vi "run.vi"(8 "error in (no error)":errorcluster, 11 "GenericExperiment in":refnum<class "ExperimentControllerDL090430DAQmxTriggered.lvclass">) -> (0 "error out":errorcluster, 3 "GenericExperiment out":refnum<class "ExperimentControllerDL090430DAQmxTriggered.lvclass">)   [LabVIEW 2010, in "ExperimentControllerDL090430DAQmxTriggered.lvclass"]
uses:
  ExperimentControllerDL090430DAQmxTriggered.lvclass
  internal_trigger_enum.ctl
  main/labview_source/controls/undock_button.ctl
  common/enumerations/top-level_component_type_enum.ctl
  state_enum.ctl
  ExperimentControllerDL090430DAQmxTriggered.lvclass/ExperimentControllerDL090430DAQmxTriggered.ctl
  main/labview_source/type_definitions/enumerations/main_trigger_enum.ctl
  GenericExperimentController/GenericExperimentController/GenericExperimentController.lvclass
  wait_for_enum.ctl
  common/classes/ErrorController/ErrorController/class_data.vi
  common/classes/ErrorController/ErrorController/ErrorController.lvclass
panel:
  in  "button:undock":T1
  in  "Tab Control":enum32{"User", "Debug", "About"}(tab)
  out "current sweep no.":i32
  out "last trigger":T2
  out "statemachine loop counter":i32
  out "last action":T2
  out "sender":T3=enum."ImagingMode"
  out "event loop error":errorcluster
  out "statemachine loop error":errorcluster
  out "finished?":bool
  out "state":T4
  # "With this experiment controller, each sweep is triggered by a TTL trigger."
  # "DL090430TriggeredExperimentController\n\nImplemented by:\nDominik Langer, University of Zurich, Switzerland\nMarcel van 't Hoff, University of Zurich, Switzerland"
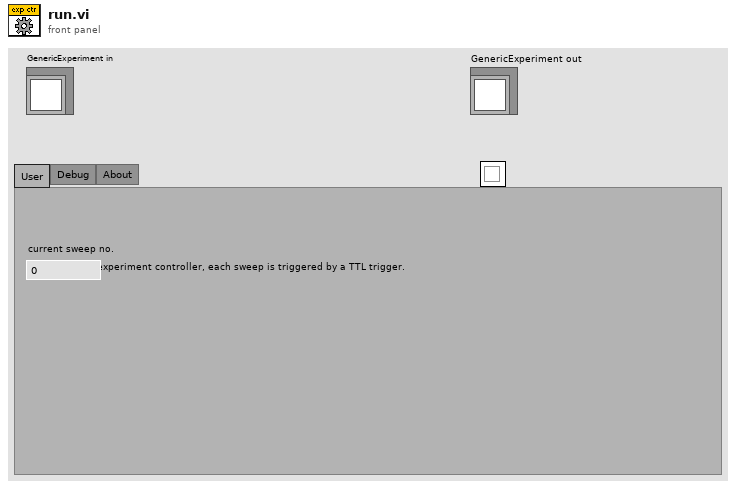
[diagram p1: front panel]
types:
  T1 = typedef "undock_button.ctl" = bool
  T2 = typedef "ExperimentControllerDL090430DAQmxTriggered.lvclass/internal_trigger_enum.ctl" = enum16{"NULL", "initialise", "terminate", "proceed", "start", "stop", "start sweep", "stop sweep"}
  T3 = typedef "top-level_component_type_enum.ctl" = enum16{"undefined", "ImagingMode", "ScanHead", "DAQ", "ImageAssembler", "Display", "DataCollection", "Analyser", "Stimulator", "ExperimentController", "Instrument", "Stage"}
  T4 = typedef "ExperimentControllerDL090430DAQmxTriggered.lvclass/state_enum.ctl" = enum16{"not in experiment", "in experiment"}
  T5 = typedef "main_trigger_enum.ctl" = enum16{"NULL", "initialise", "terminate", "start", "stop", "change objective", "change experimentController", "change imagingMode", "save notebook", "started saving", "finished saving", "expCtr ready", "expCtr missing", "imgMd ready", "imgMd missing", "scanHd ready", "scanHd missing", "DAQ ready", "DAQ missing", "imgAsm ready", "imgAsm missing", "dataColl ready", "dataColl missing", "display ready", "display missing", "analysr ready", "analysr missing", "instrmnt ready", "instrmnt missing", "stimltr ready", "stimltr missing", "stage ready", "stage missing"}
  T6 = typedef "ExperimentControllerDL090430DAQmxTriggered.lvclass/wait_for_enum.ctl" = enum16{"start", "stop"}
  T7 = typedef "ExperimentControllerDL090430DAQmxTriggered.lvclass/mode_enum.ctl" = enum16{"trigger", "gate"}
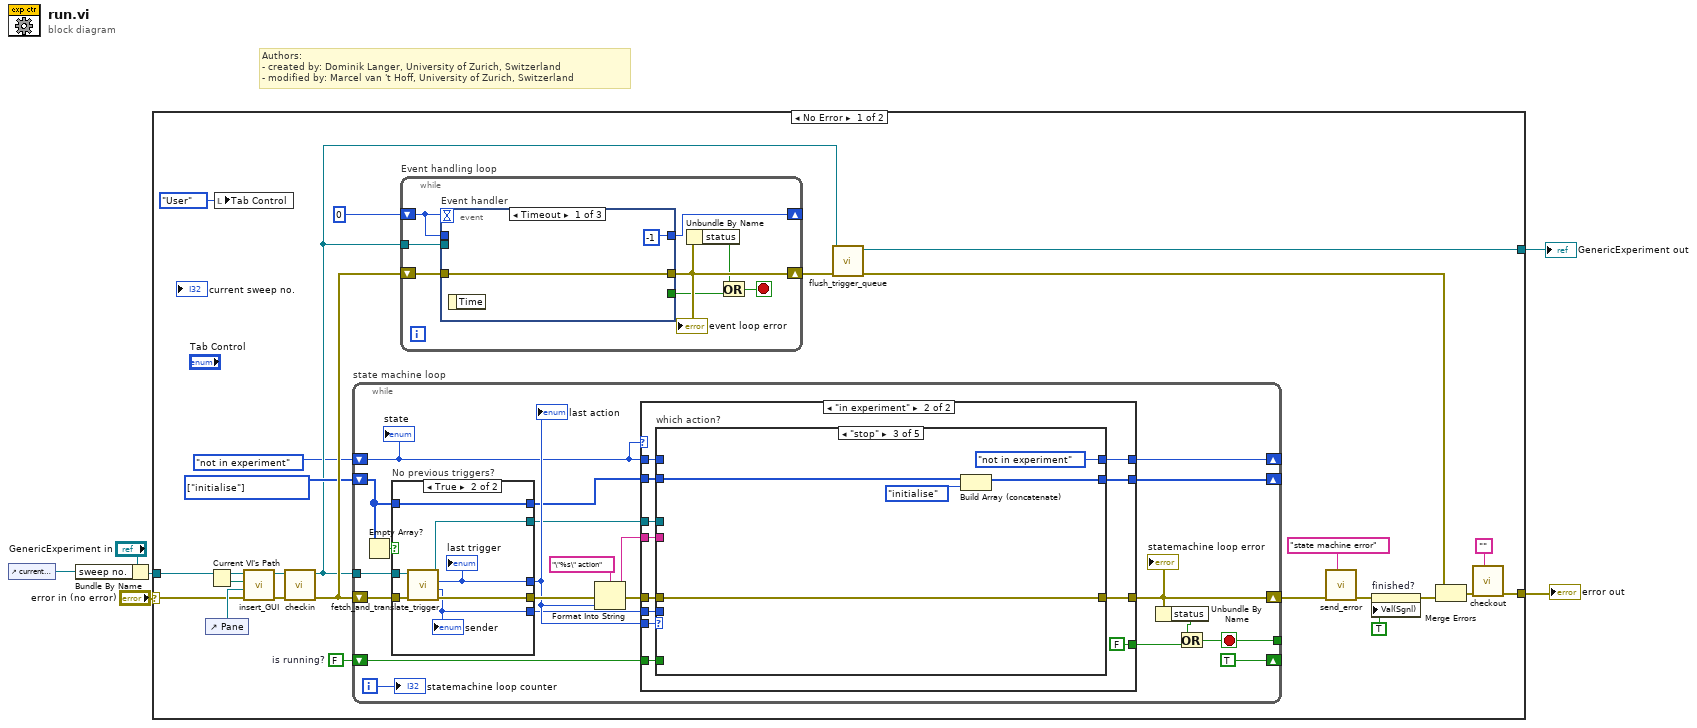
[diagram p0: block diagram]
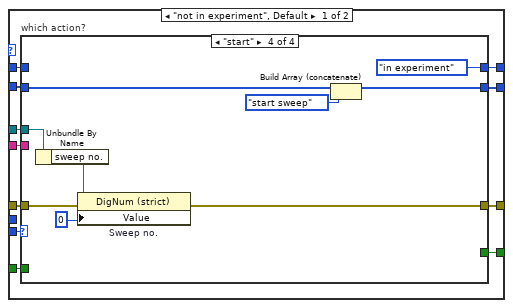
[diagram p2: hidden frame]
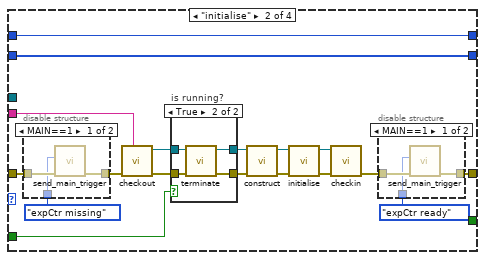
[diagram p4: hidden frame]
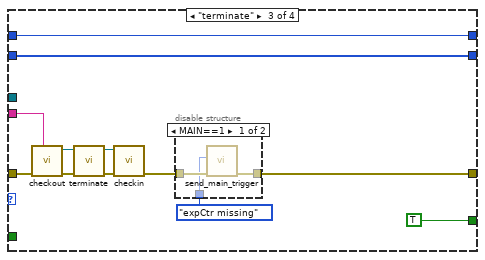
[diagram p8: hidden frame]
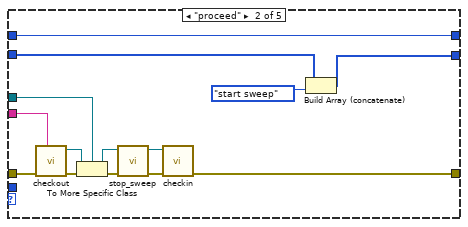
[diagram p11: hidden frame]
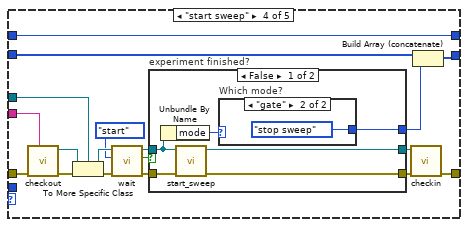
[diagram p12: hidden frame]
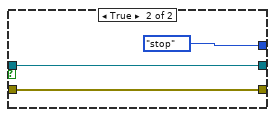
[diagram p14: hidden frame]
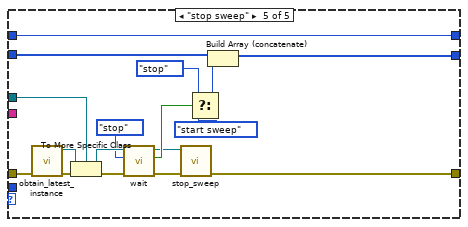
[diagram p15: hidden frame]
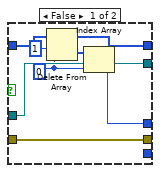
[diagram p16: hidden frame]
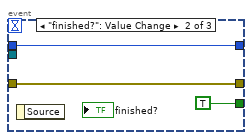
[diagram p17: hidden frame]
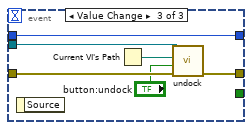
[diagram p18: hidden frame]
diagram:
  # "Authors: \n- created by: Dominik Langer, University of Zurich, Switzerland\n- modified by: Marcel van 't Hoff, University of Zurich, Switzerland"
  n1 = control-ref of="current sweep no."() -> (w1:refnum<vi>)
  n2 = Bundle By Name(cluster="GenericExperiment in", "sweep no."=w1) -> (w2:refnum<class "ExperimentControllerDL090430DAQmxTriggered.lvclass">)
  n3 = case shown="No Error" "error in (no error)" {
    selector: "error in (no error)" -> [w24 w238]
    tunnel: [w28 w238] -> w5
    tunnel: [w19 w237] -> w4
    tunnel: w2 -> [w23 w237]
    frame No Error {
      w11 = FALSE  # is running?
      w12 = T2[] [enum."initialise"] items=["NULL", "initialise", "terminate", "proceed", "start", "stop", "start sweep", "stop sweep"]
      n4 = control-ref of="Pane"() -> (w25:refnum<vi>)
      n5 = Current VI's Path() -> (path=w26:path)
      n6 = local write "Tab Control"(enum32{"User", "Debug", "About"}."User" ("Tab Control")) -> ()
      n7 = call-dynamic "insert_GUI.vi"("error in (no error)"=w24, "Pane"=w25, "VI path"=w26, "GenericComponent in"=w23) -> ("error out"=w22:errorcluster, "GenericComponent out"=w21:refnum<class "ExperimentControllerDL090430DAQmxTriggered.lvclass">)  [unwired: 6 in]
      n8 = call-dynamic "checkin.vi"("error in (no error)"=w22, "GenericExperimentController in"=w21) -> ("error out"=w13:errorcluster, "GenericExperimentController out"=w9:refnum<class "ExperimentControllerDL090430DAQmxTriggered.lvclass">)  [unwired: 8 in]
      n9 = while "state machine loop" {
        shift-right: [w37] -> w10
        shift-left: w13 -> [w52]
        shift-right: [w43] -> _
        shift-left: w12 -> [w49]
        shift-right: [TRUE ("is running?")] -> _
        shift-left: w11 -> [w40]
        tunnel: w9 -> [w51]
        tunnel: [w34] -> _
        shift-right: [w32] -> _
        shift-left: state_enum."not in experiment" ("state") -> [w31]
        i -> [w33]
        stop <- w34 stop-if-true
        n10 = Empty Array?(array=w49) -> (empty?=w50:bool)
        n11 = case "No previous triggers?" shown="True" w50 {
          tunnel: w51 -> [w210 w215]
          tunnel: w52 -> [w208 w216]
          tunnel: [w210 w214] -> w44
          tunnel: [w206 w212] -> w46
          tunnel: [_ w211] -> w38
          tunnel: [w208 w213] -> w47
          tunnel: w49 -> [w209 w217]
          tunnel: [w205 w217] -> w42
          frame False {
            w203 = 0 ("index")
            n12 = Delete From Array(array=w209, length=1, index=w203) -> (deleted portion=w207:T2[], array with subset deleted=w205:T2[])
            n13 = Index Array(array=w207, index=w203) -> (element=w206:T2)
          }
          frame True {
            n14 = call-dynamic "fetch_and_translate_trigger.vi"("error in (no error)"=w216, "ExperimentControllerDL090430DAQmxTriggered in"=w215) -> ("error out"=w213:errorcluster, "sender TLC type"=w211:T3, "statechart trigger"=w212:T2, "ExperimentControllerDL090430DAQmxTriggered out"=w214:refnum<class "ExperimentControllerDL090430DAQmxTriggered.lvclass">)  [unwired: 6 in]
            "last trigger" <- w212
            "sender" <- w211
          }
        }
        "last action" <- w46
        n15 = Format Into String(format string="\"%s\" action", error in=w47, w46) -> (resulting string=w41:string, error out=w45:errorcluster)  [unwired: 1 in]
        n16 = case shown="\"in experiment\"" w31 {
          tunnel: w46 -> [w56 w135]
          tunnel: w45 -> [w58 w134]
          tunnel: w44 -> [w60 w133]
          tunnel: [w55 w132] -> w43
          tunnel: w42 -> [w62 w131]
          tunnel: w41 -> [w61 w130]
          tunnel: w40 -> [w57 w129]
          tunnel: w38 -> [_ w128]
          tunnel: [w59 w127] -> w37
          tunnel: [w53 FALSE] -> w36
          tunnel: w31 -> [w63 w126]
          tunnel: [w54 w125] -> w32
          frame "not in experiment", Default {
            n17 = case "which action?" shown="\"start\"" w56 {
              tunnel: [w65 w76 w100 w115] -> w59
              tunnel: w58 -> [w65 w74 w104 w118]
              tunnel: w60 -> [_ _ _ w117]
              tunnel: [w66 w84 w110 w121] -> w55
              tunnel: w62 -> [w66 w84 w110 w122]
              tunnel: w61 -> [_ w79 w103 _]
              tunnel: w57 -> [_ w68 _ _]
              tunnel: [_ _ TRUE _] -> w53
              tunnel: w63 -> [w64 w67 w99 _]
              tunnel: [w64 w67 w99 state_enum."in experiment" ("state")] -> w54
              frame "NULL", Default {
              }
              frame "initialise" {
                n18 = disable-structure shown="MAIN==1" {
                  disable-tunnel: w74 -> [w93 w94]
                  disable-tunnel: [w92 w94] -> w73
                  disable-tunnel: main_trigger_enum."expCtr missing" ("trigger") -> [w91 _]
                  frame condition #0 {
                    n19 = call "send_main_trigger.vi"("error in (no error)"=w93, "trigger"=w91) -> ("error out"=w92:errorcluster)  [unwired: 9 in]
                  }
                  frame condition #1 (active) {
                  }
                }
                n20 = call "checkout.vi"("locked by?"=w79, "error in (no error)"=w73) -> ("error out"=w71:errorcluster, "GenericExperimentController out"=w72:refnum<class "GenericExperimentController.lvclass">)  [unwired: 1 in, 7 out]
                n21 = case "is running?" shown="True" w68 {
                  tunnel: w72 -> [w85 w90]
                  tunnel: w71 -> [w86 w89]
                  tunnel: [w86 w88] -> w70
                  tunnel: [w85 w87] -> w69
                  frame False {
                  }
                  frame True {
                    n22 = call-dynamic "terminate.vi"("error in (no error)"=w89, "GenericPlugin in"=w90) -> ("error out"=w88:errorcluster, "GenericPlugin out"=w87:refnum<class "GenericExperimentController.lvclass">)  [unwired: 8 out]
                  }
                }
                n23 = call-dynamic "construct.vi"("error in (no error)"=w70, "GenericPlugin in"=w69) -> ("error out"=w80:errorcluster, "GenericPlugin out"=w81:refnum<class "GenericExperimentController.lvclass">)  [unwired: 2 in, 6 out]
                n24 = call-dynamic "initialise.vi"("error in (no error)"=w80, "GenericPlugin in"=w81) -> ("error out"=w82:errorcluster, "GenericPlugin out"=w83:refnum<class "GenericExperimentController.lvclass">)  [unwired: 8 out]
                n25 = call-dynamic "checkin.vi"("error in (no error)"=w82, "GenericExperimentController in"=w83) -> ("error out"=w77:errorcluster)  [unwired: 8 in, 1 out]
                n26 = disable-structure shown="MAIN==1" {
                  disable-tunnel: w77 -> [w97 w98]
                  disable-tunnel: [w96 w98] -> w76
                  disable-tunnel: main_trigger_enum."expCtr ready" ("trigger") -> [w95 _]
                  frame condition #0 {
                    n27 = call "send_main_trigger.vi"("error in (no error)"=w97, "trigger"=w95) -> ("error out"=w96:errorcluster)  [unwired: 9 in]
                  }
                  frame condition #1 (active) {
                  }
                }
              }
              frame "terminate" {
                n28 = call "checkout.vi"("locked by?"=w103, "error in (no error)"=w104) -> ("error out"=w105:errorcluster, "GenericExperimentController out"=w106:refnum<class "GenericExperimentController.lvclass">)  [unwired: 1 in, 7 out]
                n29 = call-dynamic "terminate.vi"("error in (no error)"=w105, "GenericPlugin in"=w106) -> ("error out"=w107:errorcluster, "GenericPlugin out"=w108:refnum<class "GenericExperimentController.lvclass">)  [unwired: 8 out]
                n30 = call-dynamic "checkin.vi"("error in (no error)"=w107, "GenericExperimentController in"=w108) -> ("error out"=w101:errorcluster)  [unwired: 8 in, 1 out]
                n31 = disable-structure shown="MAIN==1" {
                  disable-tunnel: w101 -> [w113 w114]
                  disable-tunnel: [w112 w114] -> w100
                  disable-tunnel: main_trigger_enum."expCtr missing" ("trigger") -> [w111 _]
                  frame condition #0 {
                    n32 = call "send_main_trigger.vi"("error in (no error)"=w113, "trigger"=w111) -> ("error out"=w112:errorcluster)  [unwired: 9 in]
                  }
                  frame condition #1 (active) {
                  }
                }
              }
              frame "start" {
                n33 = Unbundle By Name(w117) -> ("sweep no."=w120:refnum<vi>)
                n34 = property on="Sweep no." class="DigNum (strict)"(reference=w120, error in=w118, "Value"=0) -> (error out=w115:errorcluster)  [unwired: 1 out]
                n35 = Build Array (concatenate)(w122, internal_trigger_enum."start sweep" ("internal trigger enum")) -> (w121:T2[])
              }
            }
          }
          frame "in experiment" {
            n36 = case "which action?" shown="\"stop\"" w135 {
              tunnel: [w137 w145 w153 w164 w187] -> w127
              tunnel: w134 -> [w137 w146 w153 w170 w200]
              tunnel: w133 -> [_ w143 _ w167 w199]
              tunnel: [w138 w141 w156 w173 w197] -> w132
              tunnel: w131 -> [w138 w142 w157 w175 w198]
              tunnel: w130 -> [_ w144 _ w169 _]
              tunnel: w129 -> [_ _ _ _ _]
              tunnel: w128 -> [_ _ _ _ _]
              tunnel: w126 -> [w136 w139 _ w158 w186]
              tunnel: [w136 w139 state_enum."not in experiment" ("state") w158 w186] -> w125
              frame "NULL", Default {
              }
              frame "proceed" {
                n37 = call "checkout.vi"("locked by?"=w144, "error in (no error)"=w146) -> ("error out"=w147:errorcluster, "GenericExperimentController out"=w148:refnum<class "GenericExperimentController.lvclass">)  [unwired: 1 in, 7 out]
                n38 = To More Specific Class(target class=w143, reference=w148, error in=w147) -> (specific class reference=w150:refnum<class "ExperimentControllerDL090430DAQmxTriggered.lvclass">, error out=w149:errorcluster)
                n39 = call-dynamic "stop_sweep.vi"("error in (no error)"=w149, "DL090430TriggeredExperimentController in"=w150) -> ("error out"=w151:errorcluster, "DL090430TriggeredExperimentController out"=w152:refnum<class "ExperimentControllerDL090430DAQmxTriggered.lvclass">)  [unwired: 8 out]
                n40 = call-dynamic "checkin.vi"("error in (no error)"=w151, "GenericExperimentController in"=w152) -> ("error out"=w145:errorcluster)  [unwired: 8 in, 1 out]
                n41 = Build Array (concatenate)(w142, internal_trigger_enum."start sweep" ("internal trigger enum")) -> (w141:T2[])
              }
              frame "stop" {
                n42 = Build Array (concatenate)(w157, internal_trigger_enum."initialise" ("internal trigger enum")) -> (w156:T2[])
              }
              frame "start sweep" {
                n43 = call "checkout.vi"("locked by?"=w169, "error in (no error)"=w170) -> ("error out"=w171:errorcluster, "GenericExperimentController out"=w168:refnum<class "GenericExperimentController.lvclass">)  [unwired: 1 in, 7 out]
                n44 = To More Specific Class(target class=w167, reference=w168, error in=w171) -> (specific class reference=w166:refnum<class "ExperimentControllerDL090430DAQmxTriggered.lvclass">, error out=w172:errorcluster)
                n45 = call-dynamic "wait.vi"("error in (no error)"=w172, "wait for"=wait_for_enum."start", "DL090430TriggeredExperimentController in"=w166) -> ("error out"=w160:errorcluster, "experiment finished?"=w162:bool, "DL090430TriggeredExperimentController out"=w161:refnum<class "ExperimentControllerDL090430DAQmxTriggered.lvclass">)  [unwired: 6 out]
                n46 = case "experiment finished?" shown="False" w162 {
                  tunnel: w161 -> [w177 w183]
                  tunnel: w160 -> [w181 w185]
                  tunnel: [w180 w185] -> w163
                  tunnel: [w178 internal_trigger_enum."stop" ("internal trigger enum")] -> w174
                  tunnel: [w179 w183] -> w165
                  frame False {
                    n47 = Unbundle By Name(w177) -> ("mode"=w176:T7)
                    n48 = call-dynamic "start_sweep.vi"("error in (no error)"=w181, "DL090430TriggeredExperimentController in"=w177) -> ("error out"=w180:errorcluster, "DL090430TriggeredExperimentController out"=w179:refnum<class "ExperimentControllerDL090430DAQmxTriggered.lvclass">)  [unwired: 8 out]
                    n49 = case "Which mode?" shown="\"gate\"" w176 {
                      tunnel: [_ internal_trigger_enum."stop sweep" ("internal trigger enum")] -> w178
                      frame "trigger", Default {
                      }
                      frame "gate" {
                      }
                    }
                  }
                  frame True {
                  }
                }
                n50 = call-dynamic "checkin.vi"("error in (no error)"=w163, "GenericExperimentController in"=w165) -> ("error out"=w164:errorcluster)  [unwired: 8 in, 1 out]
                n51 = Build Array (concatenate)(w175, w174) -> (w173:T2[])
              }
              frame "stop sweep" {
                n52 = call "obtain_latest_instance.vi"("error in (no error)"=w200) -> ("error out"=w201:errorcluster, "GenericExperimentController out"=w202:refnum<class "GenericExperimentController.lvclass">)  [unwired: 1 in, 8 out]
                n53 = To More Specific Class(target class=w199, reference=w202, error in=w201) -> (specific class reference=w195:refnum<class "ExperimentControllerDL090430DAQmxTriggered.lvclass">, error out=w196:errorcluster)
                n54 = call-dynamic "wait.vi"("error in (no error)"=w196, "wait for"=wait_for_enum."stop", "DL090430TriggeredExperimentController in"=w195) -> ("error out"=w188:errorcluster, "experiment finished?"=w194:bool, "DL090430TriggeredExperimentController out"=w189:refnum<class "ExperimentControllerDL090430DAQmxTriggered.lvclass">)  [unwired: 6 out]
                n55 = call-dynamic "stop_sweep.vi"("error in (no error)"=w188, "DL090430TriggeredExperimentController in"=w189) -> ("error out"=w187:errorcluster)  [unwired: 8 in, 1 out]
                n56 = Select(t=internal_trigger_enum."stop" ("internal trigger enum"), s=w194, f=internal_trigger_enum."start sweep" ("internal trigger enum")) -> (s? t:f=w191:T2)
                n57 = Build Array (concatenate)(w198, w191) -> (w197:T2[])
              }
            }
          }
        }
        "statemachine loop error" <- w37
        n58 = Unbundle By Name(w37) -> ("status"=w35:bool)
        n59 = Or(x=w35, y=w36) -> (x .or. y?=w34:bool)
        "statemachine loop counter" <- w33
        "state" <- w31
      }
      n60 = while "Event handling loop" {
        shift-right: [w224] -> _
        shift-left: 0 -> [w225]
        shift-right: [w222] -> w15
        shift-left: w13 -> [w223]
        tunnel: w9 -> [w218]
        stop <- w219 stop-if-true
        n61 = event "Event handler" shown="[0] Timeout" {
          selector: _ -> [_ _ _]
          dyn-events: _ -> [_ _ _]
          timeout: w225 -> [_ _ _]
          tunnel: [-1 w230 w236] -> w224
          tunnel: w225 -> [_ w230 w236]
          tunnel: w223 -> [w226 w228 w235]
          tunnel: [w226 w228 w234] -> w222
          tunnel: [_ TRUE _] -> w220
          tunnel: w218 -> [_ _ w231]
          event Timeout {
            n62 = event-data() -> ()  [unwired: 2 out]
          }
          event "finished?": Value Change {
            n63 = event-data() -> ()  [unwired: 2 out]
          }
          event Value Change {
            n64 = event-data() -> ()  [unwired: 2 out]
            n65 = Current VI's Path() -> (path=w232:path)
            n66 = call-dynamic "undock.vi"("error in (no error)"=w235, "undock?"="button:undock", "VI path"=w232, "GenericComponent in"=w231) -> ("error out"=w234:errorcluster)  [unwired: 6 in, 1 out]
          }
        }
        "event loop error" <- w222
        n67 = Unbundle By Name(w222) -> ("status"=w221:bool)
        n68 = Or(x=w221, y=w220) -> (x .or. y?=w219:bool)
      }
      n69 = call-dynamic "flush_trigger_queue.vi"("error in (no error)"=w15, "GenericToplevelComponent in"=w9) -> ("error out"=w20:errorcluster, "GenericToplevelComponent out"=w19:refnum<class "ExperimentControllerDL090430DAQmxTriggered.lvclass">)  [unwired: 8 in]
      n70 = call "send_error.vi"("additional message"="state machine error", "error in (no error)"=w10) -> ("error out"=w14:errorcluster)  [unwired: 9 in]
      n71 = property on="finished?" class="Bool (strict)"(error in=w14, "Val(Sgnl)"=TRUE) -> (error out=w18:errorcluster)  [unwired: 1 in, 1 out]
      n72 = Merge Errors(w20, w18) -> (w29:errorcluster)
      n73 = call "checkout.vi"("locked by?"="", "error in (no error)"=w29) -> ("error out"=w28:errorcluster)  [unwired: 1 in, 8 out]
    }
    frame Error {
    }
  }
  "error out" <- w5
  "GenericExperiment out" <- w4
